vi "COMI US Retrv Channel.vi"(6 "VarType":u32(ring) items=["VT_SHORT", "VT_FLOAT", "VT_DOUBLE"], 7 "maxNumData":i32, 9 "startCount":u32, 10 "chOrder":i32, 11 "hDevice":u32) -> (2 "function return":u32, 3 "hDevice out":u32)   [LabVIEW 2017, in "Comidll.lvlib"]
doc: "unsigned long (COMI_US_RetrvChannel) (HANDLE hDevice, int chOrder, unsigned long startCount, \n int maxNumData, void pDestBuf, TComiVarType VarType);"
uses:
  <userlib>/Comidll/Comidll.lvlib
  <userlib>/Comidll/Comidll.dll
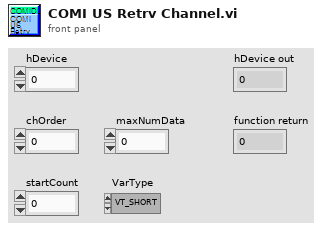
[diagram p1: front panel]
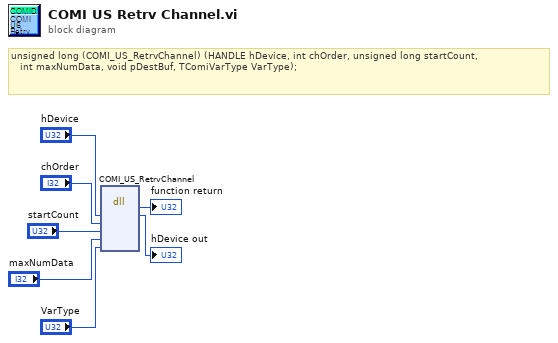
[diagram p0: block diagram]
diagram:
  # "unsigned long\t(COMI_US_RetrvChannel) (HANDLE hDevice, int chOrder, unsigned long startCount, \n\t\t\tint maxNumData, void pDestBuf, TComiVarType VarType);"
  n1 = dll-call lib="C:/Program Files/National Instruments/LabVIEW 2017/user.lib/Comidll/Comidll.*" fn="COMI_US_RetrvChannel"("hDevice"="hDevice", "chOrder"="chOrder", "startCount"="startCount", "maxNumData"="maxNumData", "VarType"="VarType") -> (→"function return":u32, "hDevice"=→"hDevice out":u32)  [unwired: 7 in, 2 out]
